vi "APS close.vi"(8 "error in (no error)":errorcluster caption="错误输入（无错误）") -> (0 "error out":errorcluster caption="错误输出", 3 "function return":i32)   [LabVIEW 2017]
doc: "I32 FNTYPE APS_close(void);"
uses:
  APS168.dll
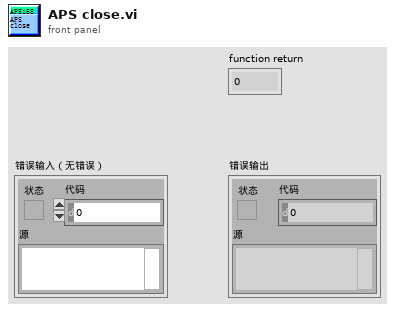
[diagram p1: front panel]
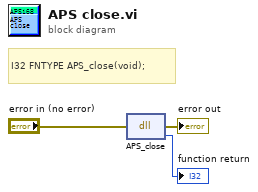
[diagram p0: block diagram]
diagram:
  # "I32 FNTYPE APS_close(void);"
  n1 = dll-call lib="PTH2Labs E迈治LV范例testSubVIsADLINKLLB运动204cAPS168.*" fn="APS_close"(error in="error in (no error)") -> (error out=→"error out":errorcluster, →"function return":i32)  [unwired: 2 in, 1 out]
